vi "GetConnected.vi"(8 "error in (no error)":errorcluster, 11 "reference in":refnum<class "Camera_Sim.lvclass">) -> (0 "error out":errorcluster, 2 "Connected":bool, 3 "reference out":refnum<class "Camera_Sim.lvclass">)   [LabVIEW 2017, in "Camera_Sim.lvclass"]
uses:
  Camera_Sim.lvclass
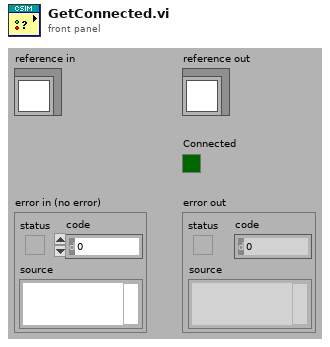
[diagram p1: front panel]
types:
  T1 = typedef "Camera_Sim.lvclass/ObjectAttributes.ctl" = cluster{"Connected":bool, "Image Out":T2, "Frame Number":u32, "Path":path}
  T2 = typedef "IMAQ Image.ctl" = refnum<image>
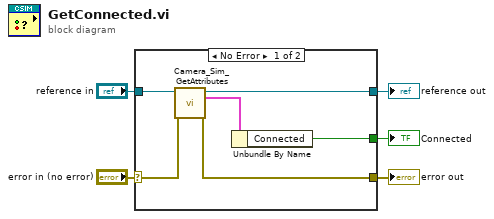
[diagram p0: block diagram]
diagram:
  n1 = case shown="No Error" "error in (no error)" {
    selector: "error in (no error)" -> [w11 w13]
    tunnel: [w9 w13] -> w4
    tunnel: [w7 w12] -> w2
    tunnel: "reference in" -> [w8 w12]
    tunnel: [w6 _] -> w1
    frame No Error {
      n2 = call "Camera_Sim_GetAttributes.vi"("reference in"=w8, "error in (no error)"=w11) -> ("reference out"=w7:refnum<class "Camera_Sim.lvclass">, "Data"=w10:T1, "error out"=w9:errorcluster)  [unwired: 10 in, 1 out]
      n3 = Unbundle By Name(w10) -> ("Connected"=w6:bool)
    }
    frame Error {
    }
  }
  "error out" <- w4
  "reference out" <- w2
  "Connected" <- w1
